vi "AMZ_S3_UriEncode String v4.vi"(9 "Encode /":bool=TRUE, 11 "Un-encoded String":string) -> (3 "UriEncoded String":string)   [LabVIEW 2015, in "LV Interface for Amazon S3.lvlib"]
uses:
  LV Interface for Amazon S3.lvlib
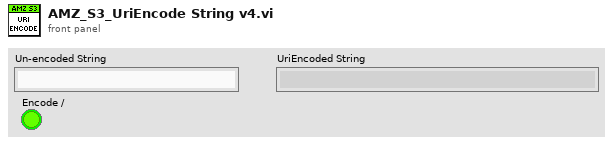
[diagram p1: front panel]
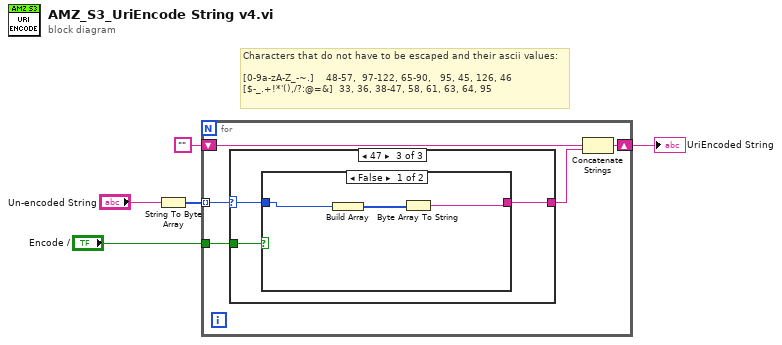
[diagram p0: block diagram]
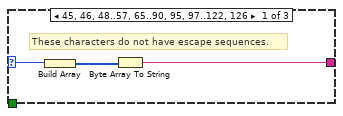
[diagram p2: hidden frame]
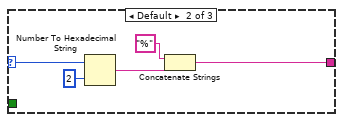
[diagram p3: hidden frame]
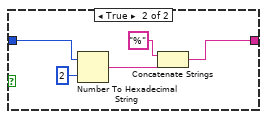
[diagram p4: hidden frame]
diagram:
  # "Characters that do not have to be escaped and their ascii values:\n\n[0-9a-zA-Z_-~.]    48-57,  97-122, 65-90,   95, 45, 126, 46 \n[$-_.+!*'(),/?:@=&]  33, 36, 38-47, 58, 61, 63, 64, 95"
  n1 = String To Byte Array(string="Un-encoded String") -> (unsigned byte array=w4:u8[])
  n2 = for {
    shift-right: [w7] -> w2
    shift-left: "" -> [w8]
    tunnel: w4 -> [w10] mode=indexing
    tunnel: "Encode /" -> [w6]
    n3 = case shown="47" w10 {
      selector: w10 -> [w13 w16 w21]
      tunnel: [w11 w15 w20] -> w9
      tunnel: w6 -> [_ _ w19]
      frame 45, 46, 48..57, 65..90, 95, 97..122, 126 {
        # "These characters do not have escape sequences."
        n4 = Build Array(w13) -> (w12:u8[])
        n5 = Byte Array To String(unsigned byte array=w12) -> (string=w11:string)
      }
      frame Default {
        n6 = Number To Hexadecimal String(1:i16 2 ("width (-)"), 2:w16) -> (0:w17:string)
        n7 = Concatenate Strings("%" ("string"), w17) -> (w15:string)
      }
      frame 47 {
        n8 = case shown="False" w19 {
          tunnel: w21 -> [w23 w25]
          tunnel: [w22 w27] -> w20
          frame False {
            n9 = Build Array(w23) -> (w24:u8[])
            n10 = Byte Array To String(unsigned byte array=w24) -> (string=w22:string)
          }
          frame True {
            n11 = Number To Hexadecimal String(1:i16 2 ("width (-)"), 2:w25) -> (0:w28:string)
            n12 = Concatenate Strings("%" ("string"), w28) -> (w27:string)
          }
        }
      }
    }
    n13 = Concatenate Strings(w8, w9) -> (w7:string)
  }
  "UriEncoded String" <- w2
